vi "Tri2NormUV.vi"(11 "TriangleFace":T1) -> (0 "v":dbl[](array[numeric]), 1 "u":dbl[](array[numeric]), 2 "Normal":dbl[](array[numeric]), 3 "TriVertex":dbl[](array[numeric]))   [LabVIEW 2014]
uses:
  TypeDefs/TriangleFace.ctl
  TypeDefs/Point3D.ctl
  <vilib>/Analysis/NI_AALPro.lvlib
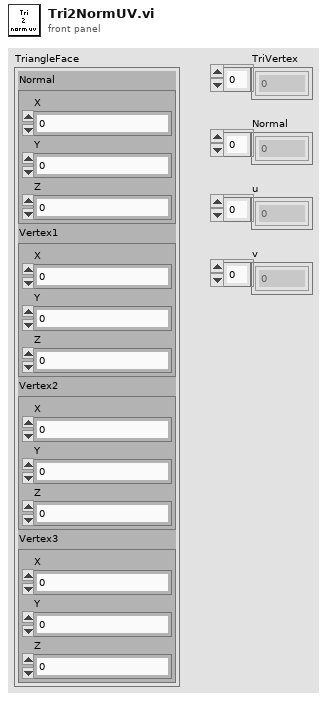
[diagram p1: front panel]
types:
  T1 = typedef "TriangleFace.ctl" = cluster{"Normal":T2, "Vertex1":T2, "Vertex2":T2, "Vertex3":T2}
  T2 = typedef "Point3D.ctl" = cluster{"X":sgl, "Y":sgl, "Z":sgl}
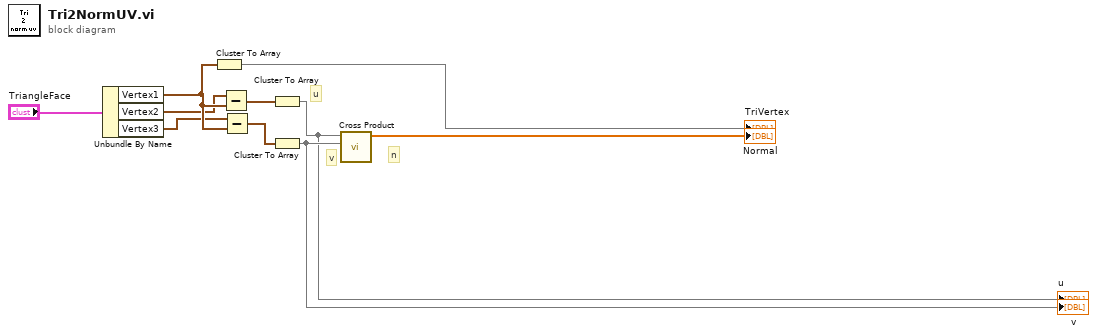
[diagram p0: block diagram]
diagram:
  # "n"
  # "v"
  # "u"
  n1 = Unbundle By Name("TriangleFace") -> ("Vertex1"=w9:T2, "Vertex2"=w7:T2, "Vertex3"=w8:T2)
  n2 = Cluster To Array(cluster=w9) -> (array=→"TriVertex":sgl[])
  n3 = Subtract(x=w7, y=w9) -> (x-y=w2:T2)
  n4 = Subtract(x=w8, y=w9) -> (x-y=w3:T2)
  n5 = Cluster To Array(cluster=w2) -> (array=w5:sgl[])
  "u" <- w5
  n6 = Cluster To Array(cluster=w3) -> (array=w6:sgl[])
  "v" <- w6
  n7 = call <vilib>:"Cross Product.vi"("B Vector"=w6, "A Vector"=w5) -> ("Cross Product"=→"Normal":dbl[])  [unwired: 8 in, 1 out]
